vi "DSF.Engine.Transfer.Get Group Offset.vi"(11 "Transfer in":refnum<class "DSF.Engine.Transfer.lvclass">) -> (2 "group offset":u64, 3 "Transfer out":refnum<class "DSF.Engine.Transfer.lvclass">)   [LabVIEW 2017, in "Data Sharing Framework Engine.lvlib" / "DSF.Engine.Transfer.lvclass"]
uses:
  DSF.Engine.Transfer.lvclass
  DSF.Engine.Transfer.lvclass/DSF.Engine.Transfer.ctl
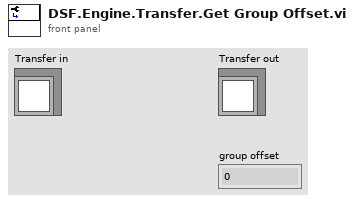
[diagram p1: front panel]
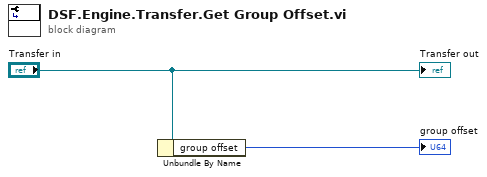
[diagram p0: block diagram]
diagram:
  n1 = Unbundle By Name("Transfer in") -> ("group offset"=→"group offset":u64)
  "Transfer out" <- "Transfer in"
